vi "ActionVIOnCompile.vi"(8 "error in (no error)":errorcluster, 11 "Device Item Ref in":T1 format="%.0x") -> (0 "error out":errorcluster)   [LabVIEW 2020, in "Ballard MIL-STD-1553 System Explorer.lvlib"]
uses:
  Ballard MIL-STD-1553 System Explorer.lvlib
  <vilib>/NI VeriStand/Custom Device API/Custom Device API.lvlib
  Includes/Ballard MIL-STD-1553 Engine.lvlibp/Engine/Implementation/Execution Unit Factory/Execution Unit Factory.lvclass
  Includes/Ballard MIL-STD-1553 Engine.lvlibp/Engine/Implementation/Shared Resources Factory/Shared Resources Factory.lvclass
  Includes/Ballard MIL-STD-1553 Engine.lvlibp/Engine/Interfaces/Execution Unit Factory/Execution Unit Factory.lvclass
  Includes/Ballard MIL-STD-1553 Engine.lvlibp/Engine/Interfaces/Shared Resources Factory/Shared Resources Factory.lvclass
  <vilib>/NI VeriStand/Custom Device API/Set Item Property (Variant).vi
  Includes/Ballard MIL-STD-1553 System Explorer.lvlibp/System Explorer/Implementation/Implementation.lvlib
  Includes/Ballard MIL-STD-1553 Engine.lvlibp/1abvi3w/vi.lib/NI VeriStand/Custom Device API/Data Reference.ctl
  Includes/Ballard MIL-STD-1553 Engine.lvlibp/1abvi3w/vi.lib/NI VeriStand/Custom Device API/Custom Device API.lvlib
  Includes/Ballard MIL-STD-1553 Engine.lvlibp/1abvi3w/vi.lib/NI VeriStand/Custom Device API/Block Data Reference.ctl
  Includes/Ballard MIL-STD-1553 Engine.lvlibp/Engine/Custom Device/Inline Execution Unit Compiled Information.ctl
  Includes/Ballard MIL-STD-1553 Engine.lvlibp/Engine/Custom Device/Custom Device.lvlib
  Includes/Ballard MIL-STD-1553 Engine.lvlibp/Engine/Custom Device/Asynchronous Execution Unit Compiled Information.ctl
  Includes/Ballard MIL-STD-1553 Engine.lvlibp/Engine/Custom Device/Compiled.Settings.ctl
  C:/Users/nitest/Desktop/Git 2020/niveristand-ballard-milStd1553-custom-device/Includes/Ballard MIL-STD-1553 Engine.lvlibp/Engine/Implementation/Execution Unit Factory/Execution Unit Factory.lvclass
  C:/Users/nitest/Desktop/Git 2020/niveristand-ballard-milStd1553-custom-device/Includes/Ballard MIL-STD-1553 Engine.lvlibp/Engine/Interfaces/Execution Unit Factory/Execution Unit Factory.lvclass
  C:/Users/nitest/Desktop/Git 2020/niveristand-ballard-milStd1553-custom-device/Includes/Ballard MIL-STD-1553 Engine.lvlibp/Engine/Implementation/Shared Resources Factory/Shared Resources Factory.lvclass
  C:/Users/nitest/Desktop/Git 2020/niveristand-ballard-milStd1553-custom-device/Includes/Ballard MIL-STD-1553 Engine.lvlibp/Engine/Interfaces/Shared Resources Factory/Shared Resources Factory.lvclass
  <vilib>/NI VeriStand/Custom Device API/Custom Device Item Ref.ctl
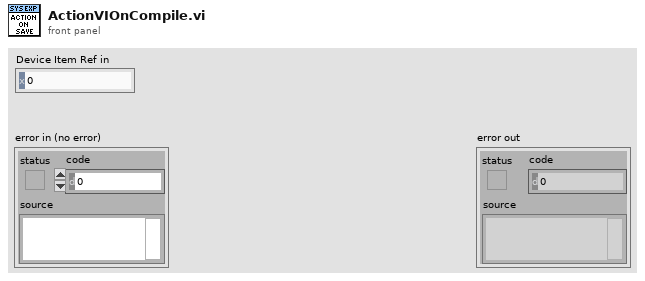
[diagram p1: front panel]
types:
  T1 = typedef "Custom Device API.lvlib/Custom Device Item Ref.ctl" = u64
  T2 = typedef "Ballard MIL-STD-1553 System Explorer.lvlibp/Custom Device API.lvlib/Custom Device Item Ref.ctl" = u64
  T3 = typedef "Ballard MIL-STD-1553 Engine.lvlibp/Custom Device.lvlib/Compiled.Settings.ctl" = cluster{"Name":string, "Inline Execution Unit Compiled Information":T4[], "Compiled Asynchronous Execution Units":cluster{"Grouped Compiled Asynchronous Execution Units":T7[]}[], "Flattened Shared Resources":string}
  T4 = typedef "Ballard MIL-STD-1553 Engine.lvlibp/Custom Device.lvlib/Inline Execution Unit Compiled Information.ctl" = cluster{"Flattened Execution Unit":string, "Incoming Buffer":dbl[], "Outgoing Buffer":dbl[], "Incoming Data References":T5[], "Outgoing Data References":T6[]}
  T5 = typedef "Ballard MIL-STD-1553 Engine.lvlibp/Custom Device API.lvlib/Data Reference.ctl" = i32
  T6 = typedef "Ballard MIL-STD-1553 Engine.lvlibp/Custom Device API.lvlib/Block Data Reference.ctl" = cluster{"Data Reference":T5, "Offset":u64, "Length":u64}
  T7 = typedef "Ballard MIL-STD-1553 Engine.lvlibp/Custom Device.lvlib/Asynchronous Execution Unit Compiled Information.ctl" = cluster{"Flattened Execution Unit":string, "Incoming Channel Group Name":string, "Outgoing Channel Group Name":string, "ReadWrite Channel Group Name":string}
  T8 = typedef "Custom Device API.lvlib/Custom Device Item Info.ctl" = cluster{"Name":string, "Is Channel":bool, "GUID":string, "Is Waveform":bool}
  T9 = typedef "Ballard MIL-STD-1553 Engine.lvlibp/Interfaces.lvlib/Execution Unit Information.ctl" = cluster{"Execution Unit":refnum<class "Execution Unit.lvclass">, "Incoming Channels":T10[], "Outgoing Channels":T10[], "ReadWrite Channels":T10[]}
  T10 = typedef "Ballard MIL-STD-1553 Engine.lvlibp/Custom Device API.lvlib/Custom Device Item Ref.ctl" = u64
  T11 = typedef "Ballard MIL-STD-1553 Shared.lvlib/Inline Execution Unit Compiled Information.ctl" = cluster{"Flattened Execution Unit":string, "Incoming Buffer":dbl[], "Outgoing Buffer":dbl[], "Incoming Data References":T12[], "Outgoing Data References":T13[]}
  T12 = typedef "Custom Device API.lvlib/Data Reference.ctl" = i32
  T13 = typedef "Custom Device API.lvlib/Block Data Reference.ctl" = cluster{"Data Reference":T12, "Offset":u64, "Length":u64}
  T14 = typedef "Ballard MIL-STD-1553 Shared.lvlib/Asynchronous Execution Unit Compiled Information.ctl" = cluster{"Flattened Execution Unit":string, "Incoming Channel Group Name":string, "Outgoing Channel Group Name":string, "ReadWrite Channel Group Name":string}
  T15 = cluster{"Compiled Grouped Asynchronous Execution Units":T14[]}[]
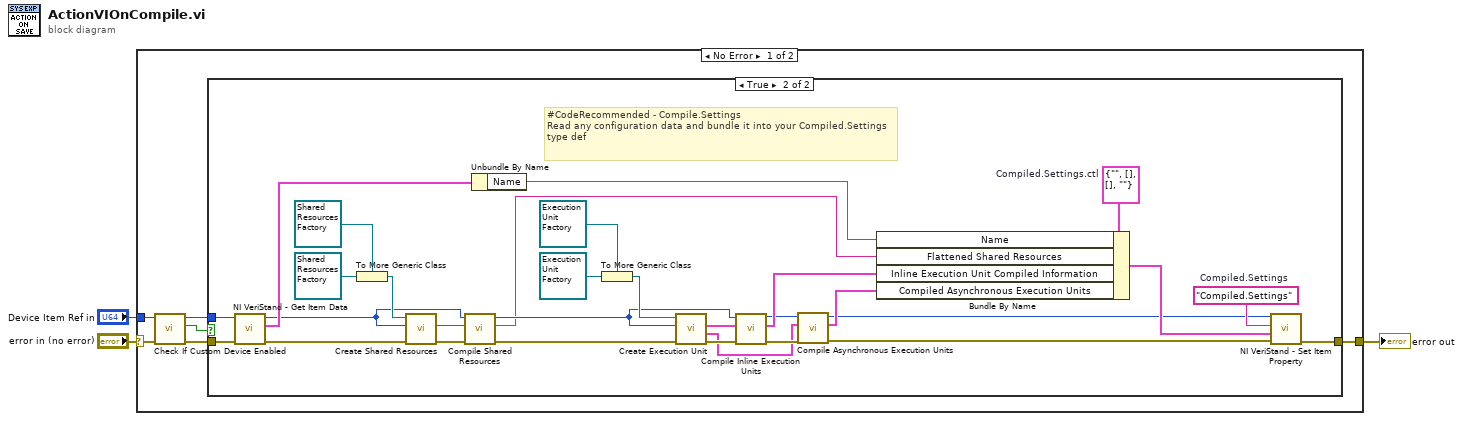
[diagram p0: block diagram]
diagram:
  n1 = case shown="No Error" "error in (no error)" {
    selector: "error in (no error)" -> [w6 w41]
    tunnel: [w9 w41] -> w2
    tunnel: "Device Item Ref in" -> [w8 _]
    frame No Error {
      n2 = call "Check If Custom Device Enabled.vi"("error in"=w6, "Ballard MIL-STD 1553 custom device in"=w8) -> ("error out"=w7:errorcluster, "Is Custom Device Enabled?"=w5:bool, "Ballard MIL-STD 1553 custom device out"=w4:T2)  [unwired: 7 in]
      n3 = case shown="True" w5 {
        tunnel: [w10 w38] -> w9
        tunnel: w7 -> [w10 w12]
        tunnel: w4 -> [_ w11]
        frame False {
          # "If custom device is not enabled, do not compile the system definition"
        }
        frame True {
          w36 = T3 {"Name"="", "Inline Execution Unit Compiled Information"=[], "Compiled Asynchronous Execution Units"=[], "Flattened Shared Resources"=""}  # Compiled.Settings.ctl
          w40 = "Compiled.Settings"  # Compiled.Settings
          # "#CodeRecommended - Compile.Settings\nRead any configuration data and bundle it into your Compiled.Settings type def"
          n4 = call <vilib>:"NI VeriStand - Get Item Data.vi"("error in (no error)"=w12, "Item Ref in"=w11) -> ("error out"=w21:errorcluster, "Item Info"=w37:T8, "Item Ref out"=w17:T1)  [unwired: 6 in, 1 out]
          n5 = To More Generic Class(target class=refnum<class "Shared Resources Factory.lvclass"> refnum ("Interfaces.lvlib:Shared Resources Factory.lvclass"), reference=refnum<class "Shared Resources Factory.lvclass"> refnum ("Implementation.lvlib:Shared Resources Factory.lvclass")) -> (generic class reference=w20:refnum<class "Shared Resources Factory.lvclass">)
          n6 = call-dynamic "Create Shared Resources.vi"("error in"=w21, "custom device ref"=w17, "shared resources factory in"=w20) -> ("error out"=w19:errorcluster, "shared resources"=w18:refnum<class "Shared Resources.lvclass">)  [unwired: 6 in, 1 out]
          n7 = call "Compile Shared Resources.vi"("error in"=w19, "shared resources"=w18, "device ref in"=w17) -> ("error out"=w15:errorcluster, "flattened shared resources"=w13:string, "device ref out"=w16:T1)  [unwired: 6 in]
          n8 = Unbundle By Name(w37) -> ("Name"=w14:string)
          n9 = To More Generic Class(target class=refnum<class "Execution Unit Factory.lvclass"> refnum ("Interfaces.lvlib:Execution Unit Factory.lvclass"), reference=refnum<class "Execution Unit Factory.lvclass"> refnum ("Implementation.lvlib:Execution Unit Factory.lvclass")) -> (generic class reference=w34:refnum<class "Execution Unit Factory.lvclass">)
          n10 = call-dynamic "Create Execution Unit.vi"("error in"=w15, "Item Ref"=w16, "Execution Unit Factory in"=w34) -> ("error out"=w35:errorcluster, "Asynchronous Execution Units"=w26:cluster{"Grouped Execution Units":T9[]}[], "Inline Execution Units"=w32:T9[])  [unwired: 5 in, 1 out]
          n11 = call "Compile Inline Execution Units.vi"("error in"=w35, "Inline Execution Units"=w32, "Device Ref in"=w16) -> ("error out"=w31:errorcluster, "Compiled Inline Execution Units"=w33:T11[], "Device Ref out"=w30:T1)  [unwired: 6 in]
          n12 = call "Compile Asynchronous Execution Units.vi"("Device Ref in"=w30, "Asynchronous Execution Units"=w26, "error in"=w31) -> ("Device Ref out"=w27:T1, "Compiled Asynchronous Execution Units"=w29:T15, "error out"=w28:errorcluster)  [unwired: 5 in]
          n13 = Bundle By Name(cluster=w36, "Name"=w14, "Flattened Shared Resources"=w13, "Inline Execution Unit Compiled Information"=w33, "Compiled Asynchronous Execution Units"=w29) -> (w39:T3)
          n14 = call-poly <vilib>:"NI VeriStand - Set Item Property.vi"("error in (no error)"=w28, "Value"=w39, "Property Name"=w40, "Item Ref in"=w27) -> ("error out"=w38:errorcluster)  [unwired: 5 in, 2 out]
        }
      }
    }
    frame Error {
    }
  }
  "error out" <- w2
